vi "Validate and Convert Path.vi"(11 "path":path) -> (3 "validated path as string":string)   [LabVIEW 2020, in "Library Commun.lvlib" / "Library Http.lvlib" / "Session.lvclass"]
uses:
  Session.lvclass
  Session.lvclass/Session.ctl
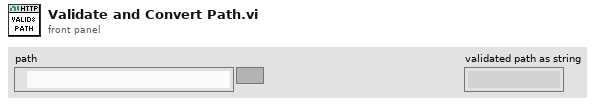
[diagram p1: front panel]
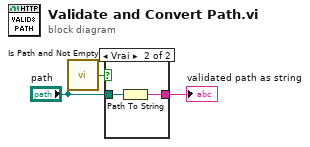
[diagram p0: block diagram]
diagram:
  n1 = call <vilib>:"Is Path and Not Empty.vi"("path"="path") -> ("Is Path and Not Empty?"=w2:bool)  [unwired: 4 in]
  n2 = case shown="Vrai" w2 {
    tunnel: [_ w4] -> w3
    tunnel: "path" -> [_ w5]
    frame False {
    }
    frame True {
      n3 = Path To String(path=w5) -> (string=w4:string)
    }
  }
  "validated path as string" <- w3
